vi "test variable set for MathCAD.vi"() -> ()   [LabVIEW 2015, in "AguaClara Library.lvlib"]
uses:
  AguaClara Library.lvlib
panel:
  out "unsigned byte array":u8[](array[numeric])
  in  "bstrName":string
  in  "Mathcad.IMathcadApplication":refnum<k7>
  in  "variable value":dbl
  out "error out":errorcluster
  in  "error in (no error)":errorcluster
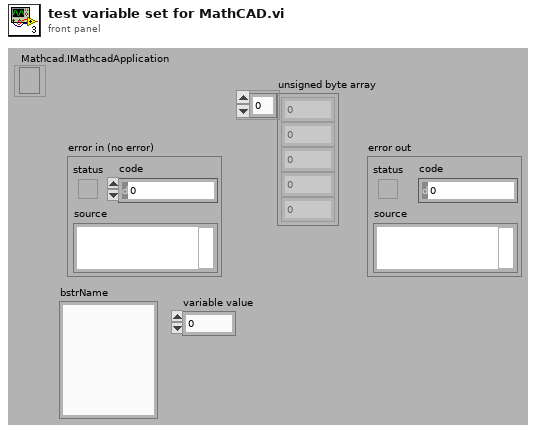
[diagram p1: front panel]
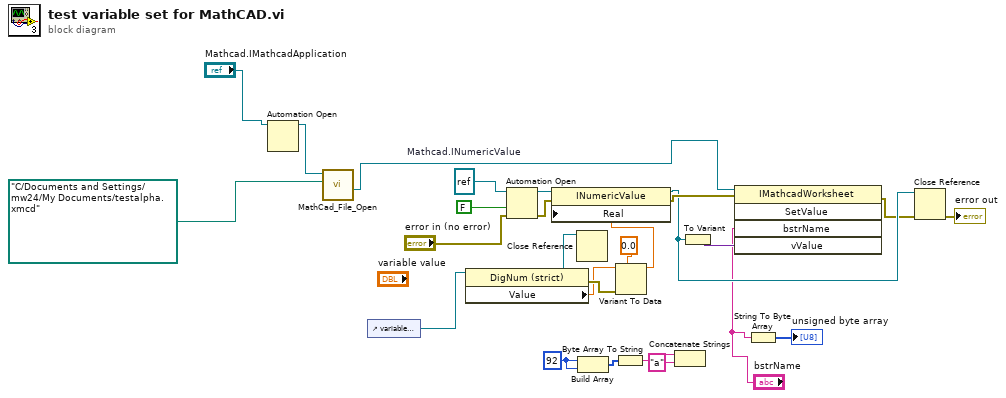
[diagram p0: block diagram]
diagram:
  w2 = 92
  w14 = refnum<k7> refnum  # Mathcad.INumericValue
  n1 = Automation Open(Automation Refnum="Mathcad.IMathcadApplication") -> (Automation Refnum=w24:refnum<k7>)  [unwired: 3 in, 1 out]
  n2 = call "MathCad_File_Open.vi"("Worksheet File"=path "C:/Documents and Settings/mw24/My Documents/testalpha.xmcd", "Mathcad.IMathcadApplication"=w24) -> ("Worksheet Reference"=w25:refnum<k7>)  [unwired: 6 in, 3 out]
  n3 = control-ref of="variable value"() -> (w9:refnum<vi>)
  n4 = property class="DigNum (strict)"(reference=w9) -> (reference out=w10:refnum<vi>, error out=w16:errorcluster, "Value"=w7:dbl)  [unwired: 1 in]
  n5 = Automation Open(error in (no error)="error in (no error)", Automation Refnum=w14, 9:FALSE ("open new instance")) -> (Automation Refnum=w21:refnum<k7>, error out=w20:errorcluster)  [unwired: 1 in]
  n6 = Close Reference(reference=w10) -> ()  [unwired: 1 in, 1 out]
  n7 = Build Array(w2, w2) -> (w5:i32[])
  n8 = Byte Array To String(unsigned byte array=w5) -> (string=w4:string)
  n9 = Variant To Data(error in=w16, type=0.0, Variant=w7) -> (data=w15:dbl)  [unwired: 1 out]
  n10 = property class="INumericValue"(reference=w21, error in=w20, "Real"=w15) -> (reference out=w18:refnum<k7>, error out=w19:errorcluster)
  n11 = Concatenate Strings(w4, "a" ("string")) -> ()  [unwired: 1 out]
  n12 = To Variant(anything=w18) -> (Variant=w8:variant)
  n13 = invoke class="IMathcadWorksheet" method="SetValue"(reference=w25, error in=w19, "bstrName"="bstrName", "vValue"=w8) -> (error out=w17:errorcluster)  [unwired: 1 in, 4 out]
  n14 = String To Byte Array(string="bstrName") -> (unsigned byte array=→"unsigned byte array":u8[])
  n15 = Close Reference(reference=w18, error in (no error)=w17) -> (error out=→"error out":errorcluster)
